vi "niusrprios Configure Rx.vi"(0 "niUsrpRio Session":T1={"FPGA Interface"=refnum, "RIO Interface Number"=0, "Data Clock Rate"=0, "FPGA Data Clock Rate"=0, "Global Settings Register Bus"=refnum, "Radio 0 Settings Register Bus"=refnum, "Radio 1 Settings Register Bus"=refnum, "Radio Settings Bus Semaphore"=refnum, "DB Queues"=[], "Characterization Data Valid?"=FALSE, "EEPROM Header"={"Checksum"=0, "Product Code"=0, "Hardware Current Version"=0, "Hardware Oldest Compatible Version"=0, "EEPROM Map Current Version"=0, "EEPROM Map Oldest Compatible Version"=0, "User Password"="", "Pointer to Factory Header"=0, "Pointer to User Header"=0, "Recommended Interval"=0, "Number of Reserved Bytes"=9, "Number of Daughterboards"=0, "Daughterboard IDs"=[], "Daughterboard Serial Numbers"=[]}, "Device Data Header"={"Checksum"=0, "Number of Channels"=0, "Number of Gain Settings"=[], "Pointer to Characterization Data"=[], "Number of Reserved Bytes"=27, "Number of Frequencies"=[]}, "EEPROM Characterization Header"={"Checksum"=0, "Date"=timestamp(0 s since 1904-01-01), "Temperature"=0.0, "Misc. Info"="", "Pointer to Device Data Header"=0, "Number of Reserved Bytes"=28}, "Characterization Data"=[], "FPGA Current Version"=0, "FPGA Oldest Compatible Version"=0, "Fixed Logic Current Version"=0, "Fixed Logic Oldest Compatible Version"=0, "FPGA Radio Settings Bus Current Version"=0, "FPGA Radio Settings Bus Oldest Compatible Version"=0, "FPGA Board Config Current Version"=0, "FPGA Board Config Oldest Compatible Version"=0, "Daughterboard Clock Rate"=0} {"Daughterboard Clock Rate" format="%#.3pHz"; "FPGA Data Clock Rate" format="%#.3pHz"; "Data Clock Rate" format="%#.3pHz"; "Characterization Data"."Frequencies [Hz]" format="%#_6p"; "EEPROM Characterization Header"."Pointer to Device Data Header" format="%x"; "EEPROM Characterization Header"."Checksum" format="%x"; "Device Data Header"."Pointer to Characterization Data" format="%x"; "Device Data Header"."Checksum" format="%x"; "EEPROM Header"."Pointer to User Header" format="%x"; "EEPROM Header"."Pointer to Factory Header" format="%x"; "EEPROM Header"."Product Code" format="%x"; "EEPROM Header"."Checksum" format="%x"}, 5 "rx config":T11={"rf enable 0"=FALSE, "rf config 0"={"antenna"="RX2", "frequency"=2000000000.0, "lo frequency"=-1.0, "level"=0.0}, "rf enable 1"=FALSE, "rf config 1"={"antenna"="RX2", "frequency"=2000000000.0, "lo frequency"=-1.0, "level"=0.0}, "transfer mode"=enum."Finite", "sample rate"=10000000.0, "number of samples"=8192, "start trigger"=enum."Immediate"} {"sample rate" format="%#.3pS/s"; "rf config 1"."level" format="%#_gdBm"; "rf config 1"."lo frequency" format="%#.3pHz"; "rf config 1"."frequency" format="%#.3pHz"; "rf config 0"."level" format="%#_gdBm"; "rf config 0"."lo frequency" format="%#.3pHz"; "rf config 0"."frequency" format="%#.3pHz"}, 11 "error in":errorcluster) -> (4 "niUsrpRio Session (out)":T1 {"Daughterboard Clock Rate" format="%#.3pHz"; "FPGA Data Clock Rate" format="%#.3pHz"; "Data Clock Rate" format="%#.3pHz"; "Characterization Data"."Frequencies [Hz]" format="%#_6p"; "EEPROM Characterization Header"."Pointer to Device Data Header" format="%x"; "EEPROM Characterization Header"."Checksum" format="%x"; "Device Data Header"."Pointer to Characterization Data" format="%x"; "Device Data Header"."Checksum" format="%x"; "EEPROM Header"."Pointer to User Header" format="%x"; "EEPROM Header"."Pointer to Factory Header" format="%x"; "EEPROM Header"."Product Code" format="%x"; "EEPROM Header"."Checksum" format="%x"}, 6 "rx.enabled channels":string[](array[string]), 8 "vertical range":dbl[](array[numeric]) format="%#.3pVpp", 14 "rx.coerced configurations":T12 {"coerced sample rates" format="%#.3pS/s"; "coerced levels" format="%#.3gdBm"; "coerced lo frequencies" format="%#.3pHz"; "coerced frequencies" format="%#.3pHz"}, 15 "error out":errorcluster)   [LabVIEW 2015]
uses:
  <instrlib>/niUsrpRio/Config/v1/Host/Public/niUsrpRio Session.ctl
  <instrlib>/_niInstr/Register Bus/v0/Host/Public/Register Bus Session.ctl
  <instrlib>/_niInstr/Register Bus/v0/Host/Private/Session Data.ctl
  <instrlib>/niUsrpRio/Config/v1/Host/Private/DB Queue Reference.ctl
  <instrlib>/niUsrpRio/Config/v1/Host/Private/Daughterboard Data.ctl
  <instrlib>/niUsrpRio/Config/v1/Host/Private/ATR state data.ctl
  <instrlib>/niUsrpRio/Config/v1/Host/Private/Antenna Configuration.ctl
  <instrlib>/niUsrpRio/Config/v1/Host/Private/CPLD Power Mode.ctl
  <instrlib>/niUsrpRio/Config/v1/Host/Public/EEPROM Header.ctl
  <instrlib>/niUsrpRio/Config/v1/Host/Public/EEPROM Device Data Header.ctl
  <instrlib>/niUsrpRio/Config/v1/Host/Public/EEPROM Characterization Header.ctl
  <instrlib>/niUsrpRio/Config/v1/Host/Public/Characterization Data.ctl
  <instrlib>/niUsrpRio/Config/v1/Host/Public/IQ Imbalance.ctl
  niusrprios Start Trigger.ctl
  niusrprios Configure Signal (Level).vi
  <instrlib>/_niInstr/Register Bus/v0/Host/niInstr Register Bus v0 Host.lvlib
  <instrlib>/niUsrpRio/Config/v1/Host/niUsrpRio Config v1 Host.lvlib
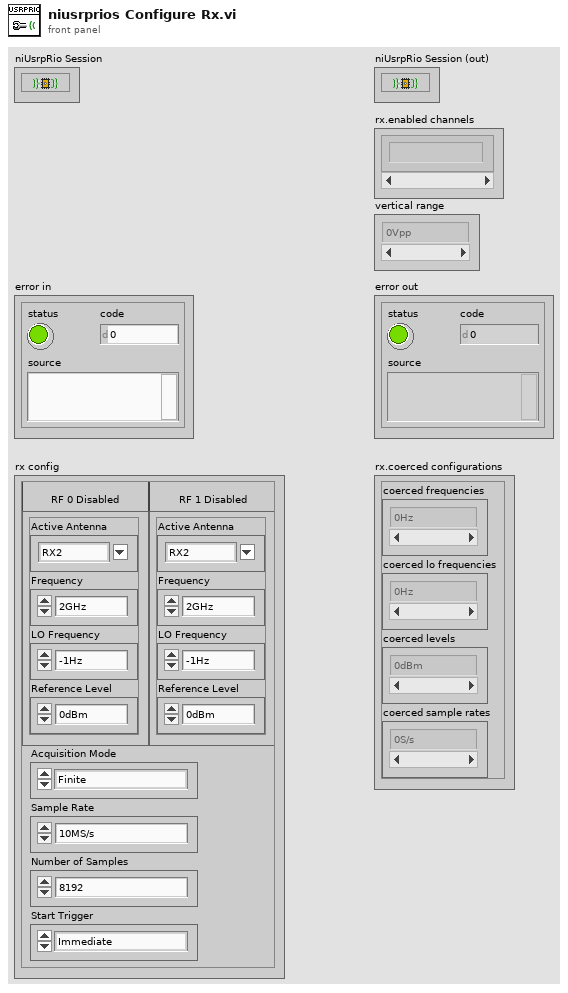
[diagram p1: front panel]
types:
  T1 = typedef "niUsrpRio Config v1 Host.lvlib/niUsrpRio Session.ctl" = cluster{"FPGA Interface":refnum<k20>, "RIO Interface Number":u32, "Data Clock Rate":u32, "FPGA Data Clock Rate":u32, "Global Settings Register Bus":T2, "Radio 0 Settings Register Bus":T2, "Radio 1 Settings Register Bus":T2, "Radio Settings Bus Semaphore":T3, "DB Queues":T4[], "Characterization Data Valid?":bool, "EEPROM Header":T5, "Device Data Header":T6, "EEPROM Characterization Header":T7, "Characterization Data":T8[], "FPGA Current Version":u32, "FPGA Oldest Compatible Version":u32, "Fixed Logic Current Version":u32, "Fixed Logic Oldest Compatible Version":u32, "FPGA Radio Settings Bus Current Version":u32, "FPGA Radio Settings Bus Oldest Compatible Version":u32, "FPGA Board Config Current Version":u32, "FPGA Board Config Oldest Compatible Version":u32, "Daughterboard Clock Rate":u32}
  T2 = typedef "niInstr Register Bus v0 Host.lvlib/Register Bus Session.ctl" = refnum<queue>
  T3 = typedef "Semaphore RefNum" = refnum<k1>
  T4 = typedef "niUsrpRio Config v1 Host.lvlib/DB Queue Reference.ctl" = refnum<queue>
  T5 = typedef "niUsrpRio Config v1 Host.lvlib/EEPROM Header.ctl" = cluster{"Checksum":u32, "Product Code":u16, "Hardware Current Version":u16, "Hardware Oldest Compatible Version":u16, "EEPROM Map Current Version":u16, "EEPROM Map Oldest Compatible Version":u16, "User Password":string, "Pointer to Factory Header":u32, "Pointer to User Header":u32, "Recommended Interval":u16, "Number of Reserved Bytes":i32, "Number of Daughterboards":u8, "Daughterboard IDs":u16[], "Daughterboard Serial Numbers":string[]}
  T6 = typedef "niUsrpRio Config v1 Host.lvlib/EEPROM Device Data Header.ctl" = cluster{"Checksum":u32, "Number of Channels":u8, "Number of Gain Settings":u16[], "Pointer to Characterization Data":u32[], "Number of Reserved Bytes":i32, "Number of Frequencies":u16[]}
  T7 = typedef "niUsrpRio Config v1 Host.lvlib/EEPROM Characterization Header.ctl" = cluster{"Checksum":u32, "Date":timestamp, "Temperature":sgl, "Misc. Info":string, "Pointer to Device Data Header":u32, "Number of Reserved Bytes":i32}
  T8 = typedef "niUsrpRio Config v1 Host.lvlib/Characterization Data.ctl" = cluster{"Gains[dB]":dbl[], "Frequencies [Hz]":dbl[], "IQ Imbalance Table":T9[], "Measured Gains[dB]":dbl[][]}
  T9 = typedef "niUsrpRio Config v1 Host.lvlib/IQ Imbalance.ctl" = cluster{"Gain Imbalance [linear]":dbl, "Phase Imbalance [radians]":dbl, "Offset":cdb}
  T10 = typedef "niusrprios Start Trigger.ctl" = enum8{"Software", "Digital Edge", "Rx Start Trigger", "Tx Start Trigger", "Immediate", "Future Time Event"}
  T11 = cluster{"rf enable 0":bool, "rf config 0":cluster{"antenna":string, "frequency":dbl, "lo frequency":dbl, "level":dbl}, "rf enable 1":bool, "rf config 1":cluster{"antenna":string, "frequency":dbl, "lo frequency":dbl, "level":dbl}, "transfer mode":enum16{"Finite", "Continuous"}, "sample rate":dbl, "number of samples":u32, "start trigger":T10}
  T12 = cluster{"coerced frequencies":dbl[], "coerced lo frequencies":dbl[], "coerced levels":dbl[], "coerced sample rates":dbl[]}
  T13 = cluster{"antenna":string, "frequency":dbl, "lo frequency":dbl, "level":dbl}
  T14 = cluster{"rf enable 0":bool, "rf config 0":cluster{"antenna":string, "frequency":dbl, "lo frequency":dbl, "level":dbl}}
  T15 = cluster{"rf enable 1":bool, "rf config 1":cluster{"antenna":string, "frequency":dbl, "lo frequency":dbl, "level":dbl}}
  T16 = cluster{"rf enable 1":bool, "rf config 1":cluster{"antenna":string, "frequency":dbl, "lo frequency":dbl, "level":dbl}}[]
  T17 = cluster{"antenna":string, "frequency":dbl, "lo frequency":dbl, "level":dbl}[]
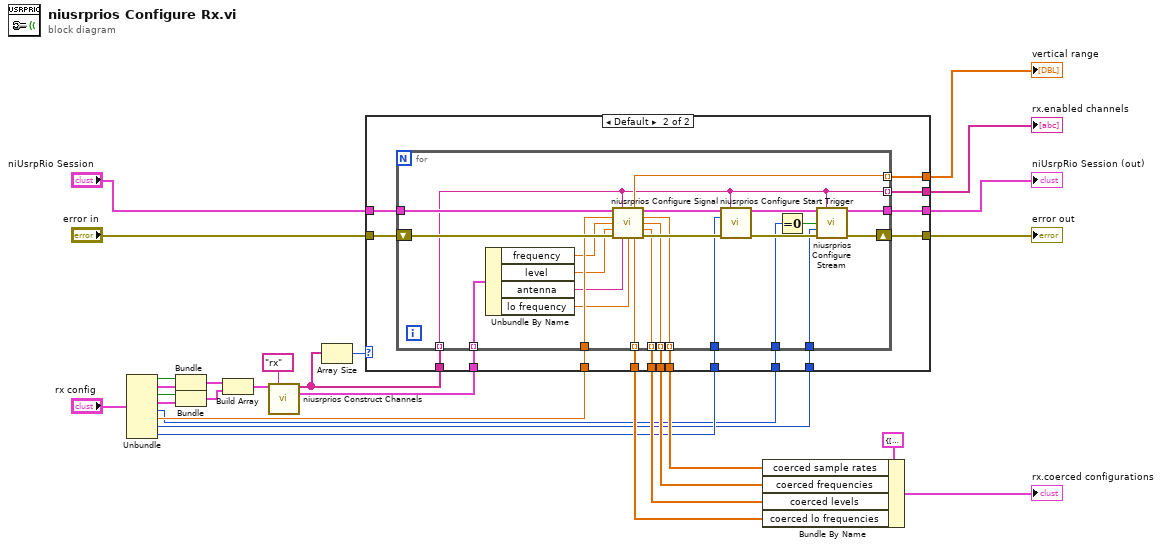
[diagram p0: block diagram]
diagram:
  n1 = Unbundle("rx config") -> ("rf enable 0"=w12:bool, "rf config 0"=w11:T13, "rf enable 1"=w10:bool, "rf config 1"=w9:T13, "transfer mode"=w1:enum16{"Finite", "Continuous"}, "sample rate"=w8:dbl, "number of samples"=w2:u32, "start trigger"=w3:T10)
  n2 = Bundle("rf enable 0"=w12, "rf config 0"=w11) -> (w15:T14)  [unwired: 1 in]
  n3 = Bundle("rf enable 1"=w10, "rf config 1"=w9) -> (w16:T15)  [unwired: 1 in]
  n4 = Build Array(w15, w16) -> (w14:T16)
  n5 = call "niusrprios Construct Channels.vi"("channel configurations"=w14, "scope"="rx") -> ("enabled channels"=w4:string[], "enabled channel configurations"=w21:T17)  [unwired: 12 in]
  n6 = Array Size(array=w4) -> (size(s)=w5:i32)
  n7 = case shown="Default" w5 {
    tunnel: [_ w46] -> w28
    tunnel: [_ w45] -> w27
    tunnel: [_ w44] -> w26
    tunnel: [_ w43] -> w25
    tunnel: [w30 w42] -> w24
    tunnel: [w29 w41] -> w23
    tunnel: w21 -> [_ w40]
    tunnel: [_ w39] -> w20
    tunnel: [_ w38] -> w17
    tunnel: w8 -> [_ w37]
    tunnel: w3 -> [_ w36]
    tunnel: w1 -> [_ w35]
    tunnel: w2 -> [_ w34]
    tunnel: "error in" -> [w29 w33]
    tunnel: "niUsrpRio Session" -> [w30 w32]
    tunnel: w4 -> [_ w31]
    frame 0 {
    }
    frame Default {
      n8 = for "channel configuration" {
        tunnel: [w67] -> w42
        shift-right: [w68] -> w41
        shift-left: w33 -> [w60]
        tunnel: w31 -> [w48] mode=indexing
        tunnel: w40 -> [w66] mode=indexing
        tunnel: [w61] -> w39 mode=indexing
        tunnel: [w65] -> w46 mode=indexing
        tunnel: [w64] -> w45 mode=indexing
        tunnel: [w63] -> w44 mode=indexing
        tunnel: [w62] -> w43 mode=indexing
        tunnel: [w48] -> w38 mode=indexing
        tunnel: w37 -> [w59]
        tunnel: w36 -> [w58]
        tunnel: w35 -> [w57]
        tunnel: w34 -> [w56]
        tunnel: w32 -> [w49]
        n9 = Unbundle By Name(w66) -> ("frequency"=w53:dbl, "level"=w52:dbl, "antenna"=w51:string, "lo frequency"=w50:dbl)
        n10 = call-poly "niusrprios Configure Signal.vi"("niUsrpRio Session"=w49, "scope"=w48, "sample rate [S/s]"=w59, "frequency [Hz]"=w53, "level [dBm]"=w52, "error in"=w60, "Active Antenna"=w51, "LO frequency [Hz]"=w50) -> ("coerced vertical range [Vpp]"=w61:dbl, "niUsrpRio Session (out)"=w54:T1, "coerced sample rate [S/s]"=w65:dbl, "coerced frequency [Hz]"=w64:dbl, "coerced level [dBm]"=w63:dbl, "coerced LO frequency [Hz]"=w62:dbl, "error out"=w69:errorcluster)  [unwired: 1 in]
        n11 = call "niusrprios Configure Start Trigger.vi"("niUsrpRio Session"=w54, "scope"=w48, "start trigger"=w58, "error in"=w69) -> ("niUsrpRio Session (out)"=w55:T1, "error out"=w70:errorcluster)  [unwired: 10 in]
        n12 = Equal To 0?(x=w57) -> (x = 0?=w47:bool)
        n13 = call "niusrprios Configure Stream.vi"("niUsrpRio Session"=w55, "scope"=w48, "number of samples is finite"=w47, "number of samples"=w56, "error in"=w70) -> ("niUsrpRio Session (out)"=w67:T1, "error out"=w68:errorcluster)  [unwired: 9 in]
      }
    }
  }
  "niUsrpRio Session (out)" <- w24
  "error out" <- w23
  "vertical range" <- w20
  "rx.enabled channels" <- w17
  n14 = Bundle By Name(cluster=T12 {"coerced frequencies"=[], "coerced lo frequencies"=[], "coerced levels"=[], "coerced sample rates"=[]} ("coerced configurations"), "coerced sample rates"=w28, "coerced frequencies"=w27, "coerced levels"=w26, "coerced lo frequencies"=w25) -> (→"rx.coerced configurations":T12)
